vi "UI.vi"() -> ()   [LabVIEW 2017]
panel:
  in  "Run":bool
  in  "Load setting":bool
  in  "stop":bool
  in  "save image":bool
  out "Runtime (ms)":u32
  in  "Save setting":bool
  out "cutting offset":dbl
  out "damaged":dbl
  out "carck":dbl
  out "glitch":dbl
  in  "output folder":path
  out "number":dbl
  in  "input folder":path
  out "display image":T1(plugin-control)
  out "NG code":dbl
  in  "NG_rules":T2
  in  "parameter":T3={"image imshow"=FALSE, "side length (mm)"=0.0, "Main Range (Threshold)"={"Lower value"=73.0, "Upper value"=255.0}, "side velocity threshold"=0.0, "Sub Range (Threshold)"={"Lower value"=73.0, "Upper value"=255.0}, "close kernel size"=0.0, "open kernel size"=0.0, "side angle offest (threshold)"=0.0}
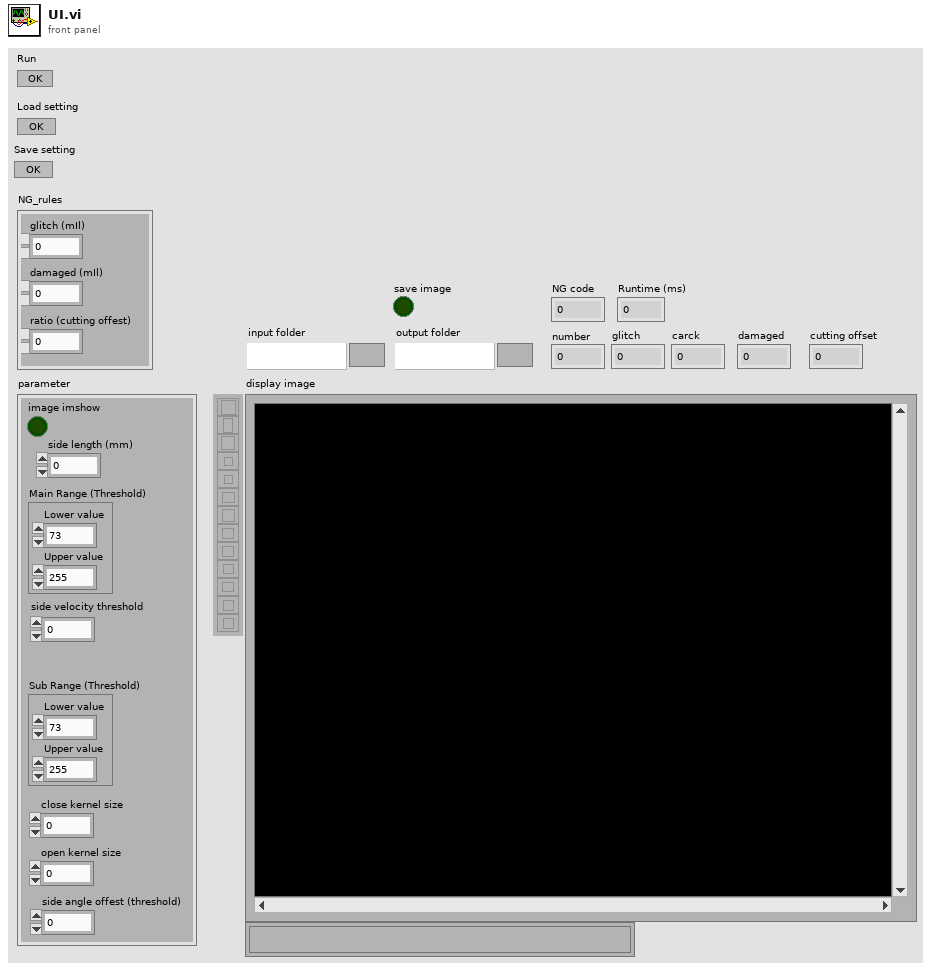
[diagram p1: front panel]
types:
  T1 = typedef "IMAQ Image.ctl" = refnum<image>
  T2 = cluster{"glitch (mIl)":dbl, "damaged (mIl)":dbl, "ratio (cutting offest)":dbl}
  T3 = cluster{"image imshow":bool, "side length (mm)":dbl, "Main Range (Threshold)":cluster{"Lower value":sgl, "Upper value":sgl}, "side velocity threshold":dbl, "Sub Range (Threshold)":cluster{"Lower value":sgl, "Upper value":sgl}, "close kernel size":dbl, "open kernel size":dbl, "side angle offest (threshold)":dbl}
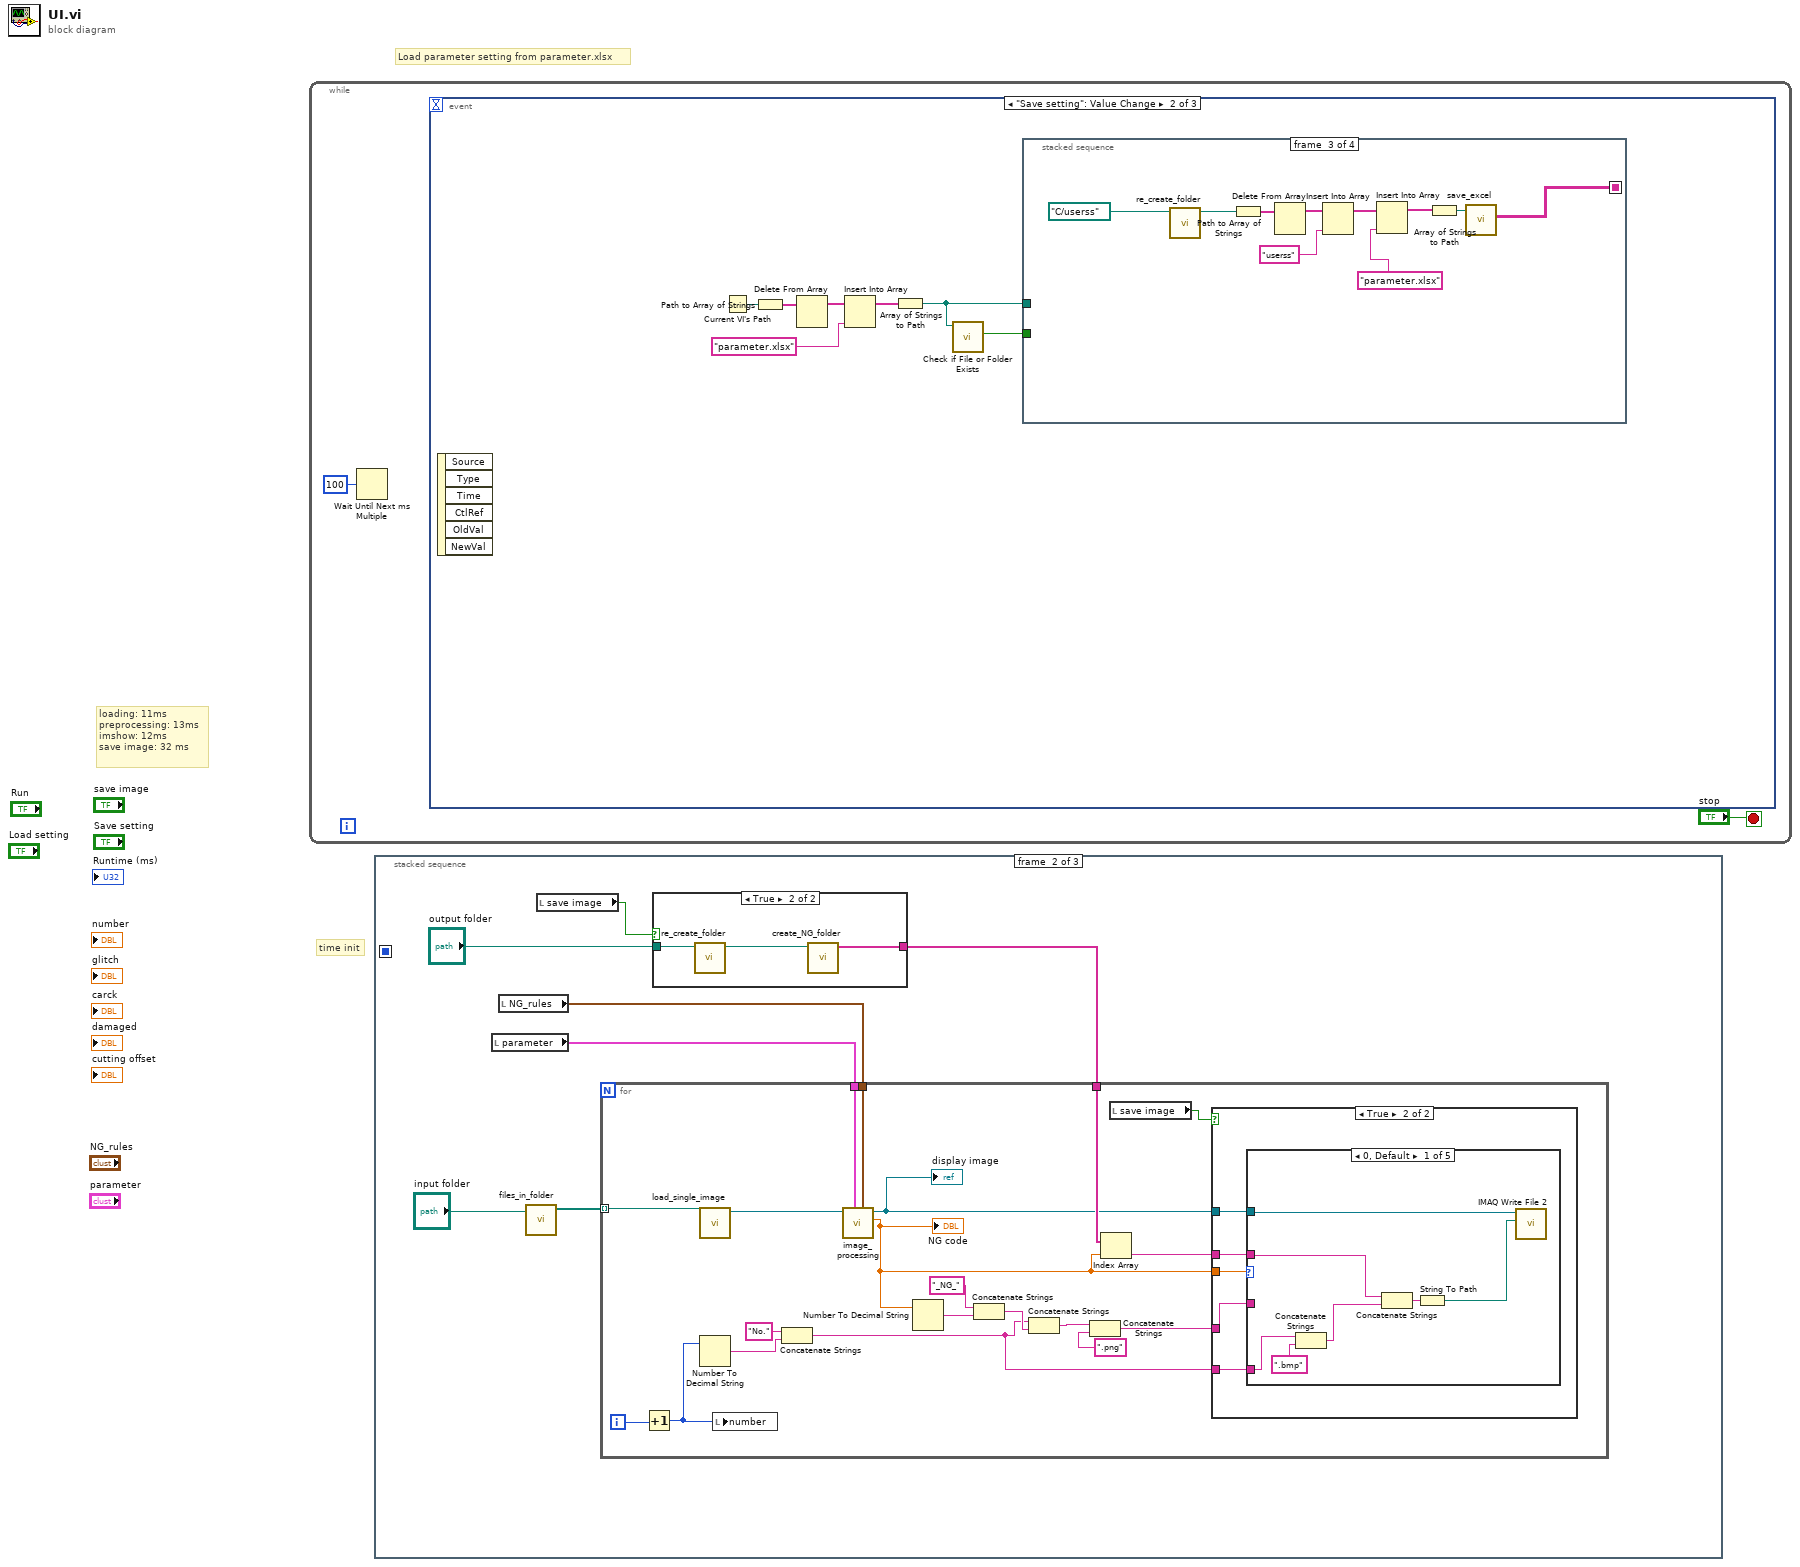
[diagram p0: block diagram]
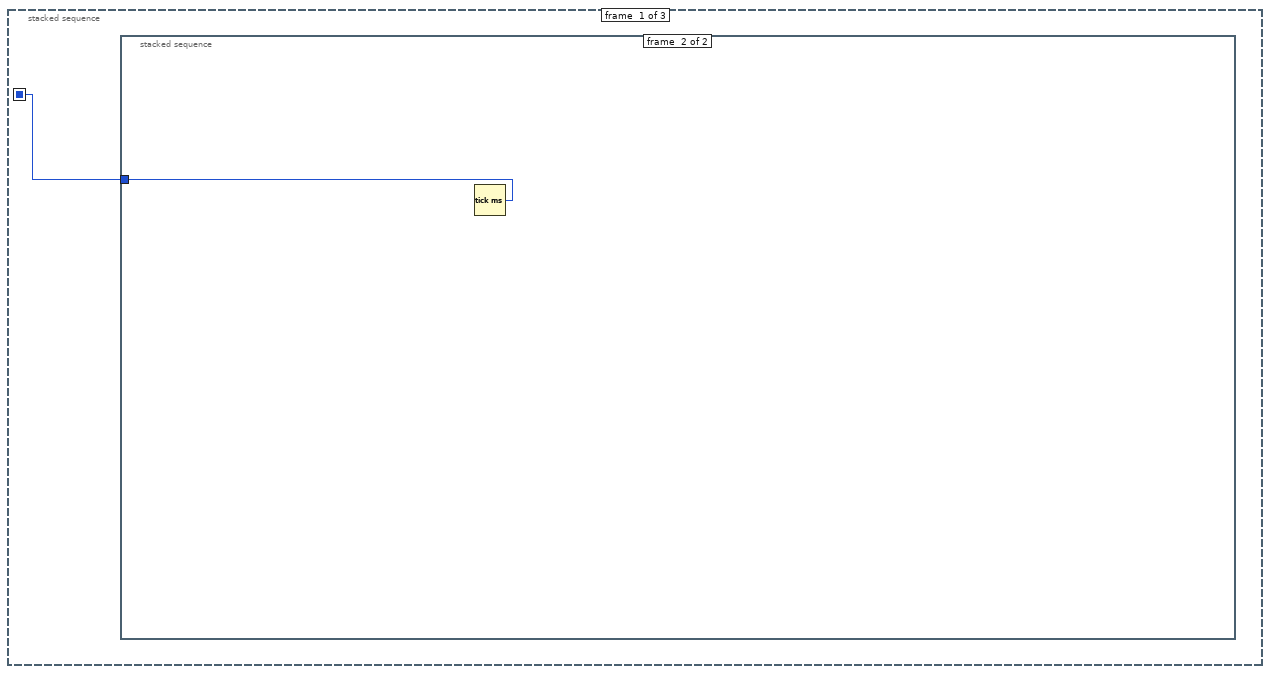
[diagram p2: hidden frame]
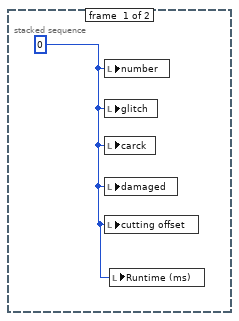
[diagram p3: hidden frame]
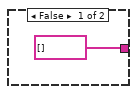
[diagram p4: hidden frame]
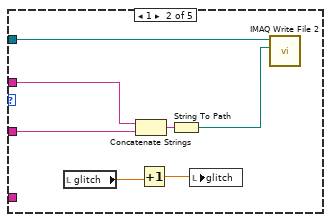
[diagram p6: hidden frame]
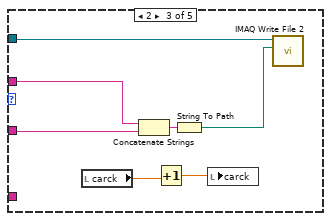
[diagram p7: hidden frame]
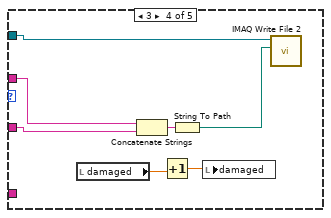
[diagram p8: hidden frame]
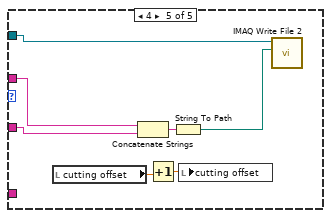
[diagram p9: hidden frame]
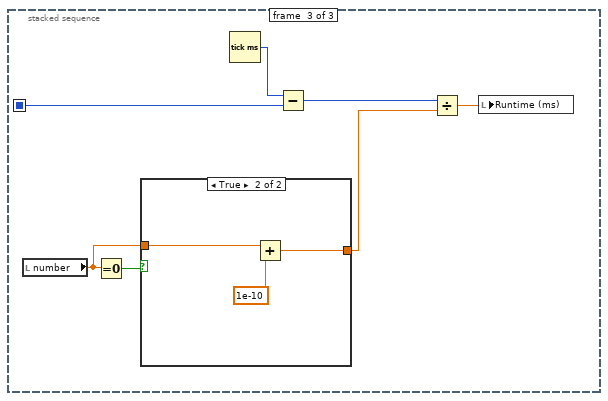
[diagram p10: hidden frame]
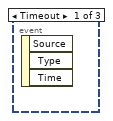
[diagram p12: hidden frame]
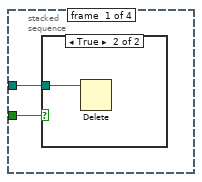
[diagram p13: hidden frame]
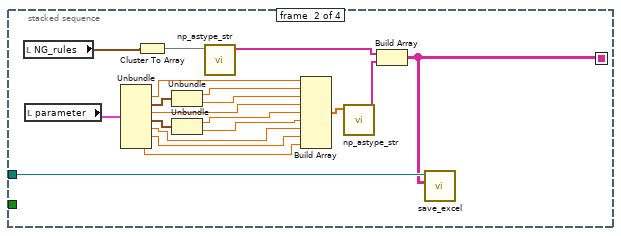
[diagram p15: hidden frame]
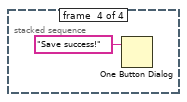
[diagram p16: hidden frame]
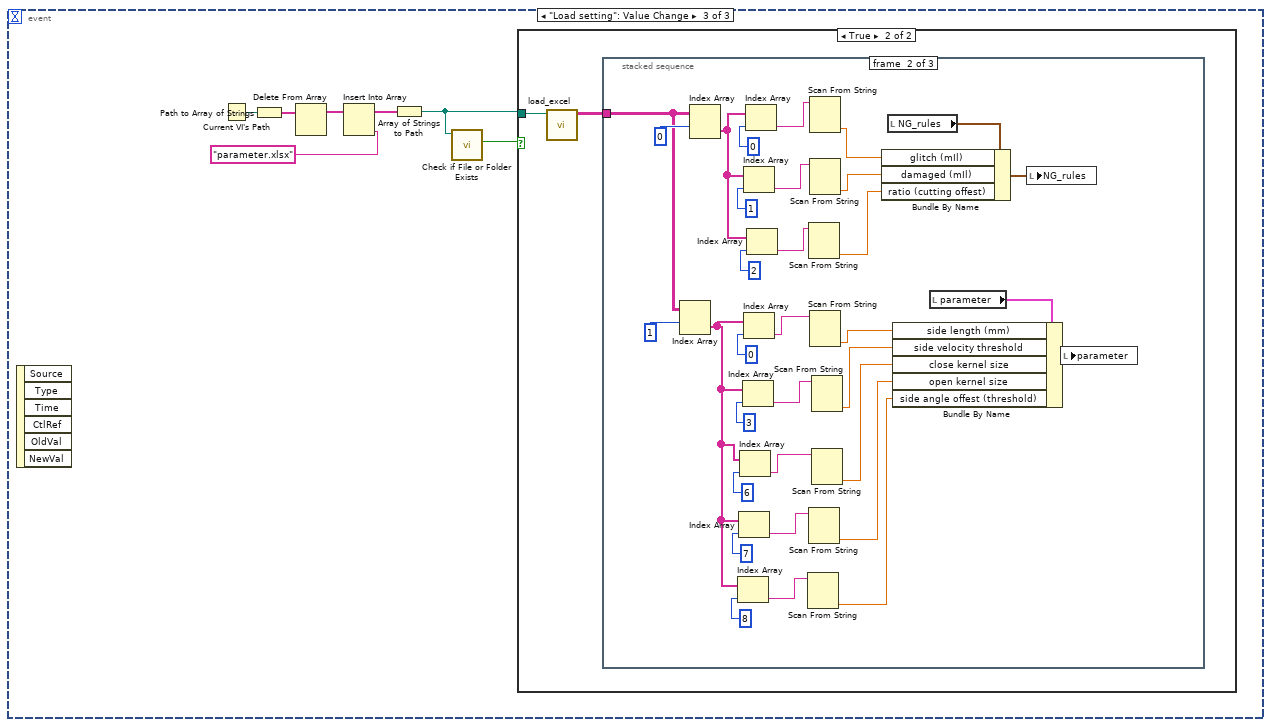
[diagram p17: hidden frame]
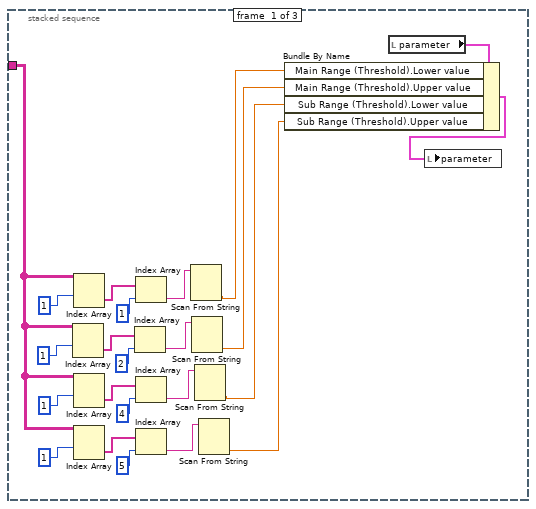
[diagram p19: hidden frame]
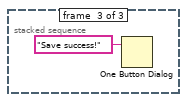
[diagram p20: hidden frame]
diagram:
  # "time init"
  # "loading: 11ms\npreprocessing: 13ms\nimshow: 12ms\nsave image: 32 ms"
  # "Load parameter setting from parameter.xlsx"
  n1 = while {
    stop <- "stop" stop-if-true
    n2 = Wait Until Next ms Multiple(millisecond multiple=u32 100) -> ()  [unwired: 1 out]
    n3 = event shown="[1] \"Save setting\": Value Change" {
      selector: _ -> [_ _ _]
      dyn-events: _ -> [_ _ _]
      timeout: _ -> [_ _ _]
      event Timeout {
        n4 = event-data() -> ()  [unwired: 1 in, 3 out]
      }
      event "Save setting": Value Change {
        n5 = event-data() -> ()  [unwired: 1 in, 6 out]
        n6 = Current VI's Path() -> (path=w7:path)
        n7 = Path to Array of Strings(0:w7) -> (2:w6:string[])  [unwired: 1 out]
        n8 = Delete From Array(array=w6) -> (array with subset deleted=w5:string[])  [unwired: 2 in, 1 out]
        n9 = Insert Into Array(array=w5, new element="parameter.xlsx" ("string")) -> (w4:string[])  [unwired: 1 in]
        n10 = Array of Strings to Path(0:w4) -> (2:w8:path)  [unwired: 1 in]
        n11 = call <vilib>:"Check if File or Folder Exists.vi"("path"=w8) -> ("file or folder exists?"=w9:bool)  [unwired: 8 in, 2 out]
        n12 = stacked-sequence {
          seq-local: [_ w13 _ _] -> [_ _ w41 _]
          tunnel: w8 -> [w11 w18 _ _]
          tunnel: w9 -> [w10 _ _ _]
          frame #0 {
            n13 = case shown="True" w10 {
              tunnel: w11 -> [_ w12]
              frame False {
              }
              frame True {
                n14 = Delete(path (use dialog)=w12) -> ()  [unwired: 4 in, 3 out]
              }
            }
          }
          frame #1 {
            n15 = local read "NG_rules"() -> (w21:T2)
            n16 = local read "parameter"() -> (w31:T3)
            n17 = Unbundle(w31) -> ("side length (mm)"=w28:dbl, "Main Range (Threshold)"=w29:cluster{"Lower value":sgl, "Upper value":sgl}, "side velocity threshold"=w25:dbl, "Sub Range (Threshold)"=w30:cluster{"Lower value":sgl, "Upper value":sgl}, "close kernel size"=w22:dbl, "open kernel size"=w15:dbl, "side angle offest (threshold)"=w14:dbl)  [unwired: 1 out]
            n18 = Cluster To Array(cluster=w21) -> (array=w20:dbl[])
            n19 = Unbundle(w29) -> ("Lower value"=w27:sgl, "Upper value"=w26:sgl)
            n20 = Unbundle(w30) -> ("Lower value"=w24:sgl, "Upper value"=w23:sgl)
            n21 = call "np_astype_str.vi"("NG_rules"=w20) -> ("Array"=w19:string[])  [unwired: 10 in]
            n22 = Build Array(w28, w27, w26, w25, w24, w23, w22, w15, w14) -> (w17:dbl[])
            n23 = call "np_astype_str.vi"("NG_rules"=w17) -> ("Array"=w16:string[])  [unwired: 10 in]
            n24 = Build Array(w19, w16) -> (w13:string[][])
            n25 = call "save_excel.vi"("data in"=w13, "Path"=w18) -> ()  [unwired: 10 in]
          }
          frame #2 {
            n26 = call "re_create_folder.vi"("output folder in"=path "C:/userss") -> ("output folder out"=w36:path)  [unwired: 10 in]
            n27 = Path to Array of Strings(0:w36) -> (2:w39:string[])  [unwired: 1 out]
            n28 = Delete From Array(array=w39) -> (array with subset deleted=w38:string[])  [unwired: 2 in, 1 out]
            n29 = Insert Into Array(array=w38, new element="userss" ("string")) -> (w34:string[])  [unwired: 1 in]
            n30 = Insert Into Array(array=w34, new element="parameter.xlsx" ("string")) -> (w33:string[])  [unwired: 1 in]
            n31 = Array of Strings to Path(0:w33) -> (2:w35:path)  [unwired: 1 in]
            n32 = call "save_excel.vi"("data in"=w41, "Path"=w35) -> ()  [unwired: 10 in]
          }
          frame #3 {
            n33 = One Button Dialog(message="Save success!") -> ()  [unwired: 1 in, 1 out]
          }
        }
      }
      event "Load setting": Value Change {
        n34 = event-data() -> ()  [unwired: 1 in, 6 out]
        n35 = Current VI's Path() -> (path=w46:path)
        n36 = Path to Array of Strings(0:w46) -> (2:w47:string[])  [unwired: 1 out]
        n37 = Delete From Array(array=w47) -> (array with subset deleted=w48:string[])  [unwired: 2 in, 1 out]
        n38 = Insert Into Array(array=w48, new element="parameter.xlsx" ("string")) -> (w49:string[])  [unwired: 1 in]
        n39 = Array of Strings to Path(0:w49) -> (2:w45:path)  [unwired: 1 in]
        n40 = call <vilib>:"Check if File or Folder Exists.vi"("path"=w45) -> ("file or folder exists?"=w44:bool)  [unwired: 8 in, 2 out]
        n41 = case shown="True" w44 {
          tunnel: w45 -> [_ w51]
          frame False {
          }
          frame True {
            n42 = call "load_excel.vi"("Path"=w51) -> ("data"=w50:string[][])  [unwired: 10 in]
            n43 = stacked-sequence {
              tunnel: w50 -> [w60 w99 _]
              frame #0 {
                n44 = Index Array(array=w60, index (row)=1) -> (element=w74:string[])  [unwired: 1 in]
                n45 = Index Array(array=w60, index (row)=1) -> (element=w61:string[])  [unwired: 1 in]
                n46 = Index Array(array=w60, index (row)=1) -> (element=w67:string[])  [unwired: 1 in]
                n47 = Index Array(array=w60, index (row)=1) -> (element=w66:string[])  [unwired: 1 in]
                n48 = Index Array(array=w74, index=2 ("index (row)")) -> (element=w55:string)
                n49 = Index Array(array=w61, index=1 ("index (row)")) -> (element=w54:string)
                n50 = Index Array(array=w67, index=4 ("index (row)")) -> (element=w53:string)
                n51 = Index Array(array=w66, index=5 ("index (row)")) -> (element=w52:string)
                n52 = Scan From String(input string=w54) -> (output 1=w59:dbl)  [unwired: 4 in, 3 out]
                n53 = Scan From String(input string=w55) -> (output 1=w58:dbl)  [unwired: 4 in, 3 out]
                n54 = Scan From String(input string=w53) -> (output 1=w57:dbl)  [unwired: 4 in, 3 out]
                n55 = Scan From String(input string=w52) -> (output 1=w56:dbl)  [unwired: 4 in, 3 out]
                n56 = local read "parameter"() -> (w72:T3)
                n57 = Bundle By Name(cluster=w72, "Main Range (Threshold).Lower value"=w59, "Main Range (Threshold).Upper value"=w58, "Sub Range (Threshold).Lower value"=w57, "Sub Range (Threshold).Upper value"=w56) -> (w71:T3)
                n58 = local write "parameter"(w71) -> ()
              }
              frame #1 {
                n59 = Index Array(array=w99, index (row)=1) -> (element=w75:string[])  [unwired: 1 in]
                n60 = Index Array(array=w99, index (row)=0) -> (element=w101:string[])  [unwired: 1 in]
                n61 = Index Array(array=w75, index=8 ("index (row)")) -> (element=w78:string)
                n62 = Index Array(array=w75, index=7 ("index (row)")) -> (element=w85:string)
                n63 = Index Array(array=w75, index=6 ("index (row)")) -> (element=w86:string)
                n64 = Index Array(array=w75, index=3 ("index (row)")) -> (element=w87:string)
                n65 = Index Array(array=w101, index=1 ("index (row)")) -> (element=w90:string)
                n66 = Index Array(array=w75, index=0 ("index (row)")) -> (element=w88:string)
                n67 = Index Array(array=w101, index=0 ("index (row)")) -> (element=w91:string)
                n68 = Index Array(array=w101, index=2 ("index (row)")) -> (element=w89:string)
                n69 = Scan From String(input string=w78) -> (output 1=w76:dbl)  [unwired: 4 in, 3 out]
                n70 = Scan From String(input string=w89) -> (output 1=w83:dbl)  [unwired: 4 in, 3 out]
                n71 = Scan From String(input string=w85) -> (output 1=w79:dbl)  [unwired: 4 in, 3 out]
                n72 = Scan From String(input string=w91) -> (output 1=w92:dbl)  [unwired: 4 in, 3 out]
                n73 = Scan From String(input string=w90) -> (output 1=w84:dbl)  [unwired: 4 in, 3 out]
                n74 = Scan From String(input string=w88) -> (output 1=w82:dbl)  [unwired: 4 in, 3 out]
                n75 = Scan From String(input string=w87) -> (output 1=w81:dbl)  [unwired: 4 in, 3 out]
                n76 = Scan From String(input string=w86) -> (output 1=w80:dbl)  [unwired: 4 in, 3 out]
                n77 = local read "NG_rules"() -> (w102:T2)
                n78 = Bundle By Name(cluster=w102, "glitch (mIl)"=w92, "damaged (mIl)"=w84, "ratio (cutting offest)"=w83) -> (w105:T2)
                n79 = local read "parameter"() -> (w93:T3)
                n80 = Bundle By Name(cluster=w93, "side length (mm)"=w82, "side velocity threshold"=w81, "close kernel size"=w80, "open kernel size"=w79, "side angle offest (threshold)"=w76) -> (w97:T3)
                n81 = local write "NG_rules"(w105) -> ()
                n82 = local write "parameter"(w97) -> ()
              }
              frame #2 {
                n83 = One Button Dialog(message="Save success!") -> ()  [unwired: 1 in, 1 out]
              }
            }
          }
        }
      }
    }
  }
  n84 = stacked-sequence {
    seq-local: [w109 _ _] -> [_ _ w188]
    frame #0 {
      n85 = stacked-sequence {
        tunnel: [_ w111] -> w109
        frame #0 {
          w110 = 0
          n86 = local write "number"(w110) -> ()
          n87 = local write "glitch"(w110) -> ()
          n88 = local write "carck"(w110) -> ()
          n89 = local write "damaged"(w110) -> ()
          n90 = local write "cutting offset"(w110) -> ()
          n91 = local write "Runtime (ms)"(w110) -> ()
        }
        frame #1 {
          n92 = Tick Count (ms)() -> (millisecond timer value=w111:u32)
        }
      }
    }
    frame #1 {
      n93 = local read "parameter"() -> (w114:T3)
      n94 = local read "NG_rules"() -> (w113:T2)
      n95 = call "files_in_folder.vi"("folder path"="input folder") -> ("Array"=w116:path[])  [unwired: 10 in]
      n96 = local read "save image"() -> (w112:bool)
      n97 = case shown="True" w112 {
        tunnel: "output folder" -> [_ w122]
        tunnel: [string[] [] ("NG folder array") w120] -> w115
        frame False {
        }
        frame True {
          n98 = call "re_create_folder.vi"("output folder in"=w122) -> ("output folder out"=w121:path)  [unwired: 10 in]
          n99 = call "create_NG_folder.vi"("output folder in"=w121) -> ("NG folder array"=w120:string[])  [unwired: 10 in]
        }
      }
      n100 = for {
        tunnel: w113 -> [w142]
        tunnel: w114 -> [w123]
        tunnel: w116 -> [w140] mode=indexing
        tunnel: w115 -> [w129]
        i -> [w137]
        n101 = Increment(x=w137) -> (x+1=w130:i32)
        n102 = call "load_single_image.vi"("Path"=w140) -> ("Refnum out"=w141:T1)  [unwired: 10 in]
        n103 = Number To Decimal String(number=w130) -> (decimal integer string=w133:string)  [unwired: 1 in]
        n104 = local write "number"(w130) -> ()
        n105 = Concatenate Strings("No." ("string"), w133) -> (w126:string)
        n106 = call "image_processing.vi"("NG_rules"=w142, "parameter"=w123, "image"=w141) -> ("NG code"=w128:dbl, "display image"=w124:T1)  [unwired: 6 in, 1 out]
        "NG code" <- w128
        "display image" <- w124
        n107 = Number To Decimal String(number=w128) -> (decimal integer string=w136:string)  [unwired: 1 in]
        n108 = Concatenate Strings("_NG_" ("string"), w136) -> (w131:string)
        n109 = Concatenate Strings(w126, w131) -> (w132:string)
        n110 = Concatenate Strings(w132, ".png" ("string")) -> (w138:string)
        n111 = Index Array(array=w129, index=w128) -> (element=w127:string)
        n112 = local read "save image"() -> (w125:bool)
        n113 = case shown="True" w125 {
          tunnel: w124 -> [_ w147]
          tunnel: w138 -> [_ w146]
          tunnel: w128 -> [_ w143]
          tunnel: w127 -> [_ w145]
          tunnel: w126 -> [_ w144]
          frame False {
          }
          frame True {
            n114 = case shown="0, Default" w143 {
              tunnel: w147 -> [w152 w161 w165 w173 w180]
              tunnel: w146 -> [_ w158 w166 w172 w179]
              tunnel: w145 -> [w151 w155 w162 w169 w176]
              tunnel: w144 -> [w150 _ _ _ _]
              frame 0, Default {
                n115 = Concatenate Strings(w150, ".bmp" ("string")) -> (w148:string)
                n116 = Concatenate Strings(w151, w148) -> (w153:string)
                n117 = String To Path(string=w153) -> (path=w154:path)
                n118 = call-poly "IMAQ Write File 2"("File Path"=w154, "Image"=w152) -> ()  [unwired: 8 in, 2 out]
              }
              frame 1 {
                n119 = local read "glitch"() -> (w157:dbl)
                n120 = Concatenate Strings(w155, w158) -> (w159:string)
                n121 = Increment(x=w157) -> (x+1=w156:dbl)
                n122 = String To Path(string=w159) -> (path=w160:path)
                n123 = local write "glitch"(w156) -> ()
                n124 = call-poly "IMAQ Write File 2"("File Path"=w160, "Image"=w161) -> ()  [unwired: 8 in, 2 out]
              }
              frame 2 {
                n125 = local read "carck"() -> (w164:dbl)
                n126 = Concatenate Strings(w162, w166) -> (w167:string)
                n127 = Increment(x=w164) -> (x+1=w163:dbl)
                n128 = String To Path(string=w167) -> (path=w168:path)
                n129 = local write "carck"(w163) -> ()
                n130 = call-poly "IMAQ Write File 2"("File Path"=w168, "Image"=w165) -> ()  [unwired: 8 in, 2 out]
              }
              frame 3 {
                n131 = local read "damaged"() -> (w171:dbl)
                n132 = Concatenate Strings(w169, w172) -> (w174:string)
                n133 = Increment(x=w171) -> (x+1=w170:dbl)
                n134 = String To Path(string=w174) -> (path=w175:path)
                n135 = local write "damaged"(w170) -> ()
                n136 = call-poly "IMAQ Write File 2"("File Path"=w175, "Image"=w173) -> ()  [unwired: 8 in, 2 out]
              }
              frame 4 {
                n137 = local read "cutting offset"() -> (w178:dbl)
                n138 = Concatenate Strings(w176, w179) -> (w181:string)
                n139 = Increment(x=w178) -> (x+1=w177:dbl)
                n140 = String To Path(string=w181) -> (path=w182:path)
                n141 = local write "cutting offset"(w177) -> ()
                n142 = call-poly "IMAQ Write File 2"("File Path"=w182, "Image"=w180) -> ()  [unwired: 8 in, 2 out]
              }
            }
          }
        }
      }
    }
    frame #2 {
      n143 = local read "number"() -> (w184:dbl)
      n144 = Equal To 0?(x=w184) -> (x = 0?=w186:bool)
      n145 = case shown="True" w186 {
        tunnel: [w190 w192] -> w185
        tunnel: w184 -> [w190 w191]
        frame False {
        }
        frame True {
          n146 = Add(x=w191, y=1e-10) -> (x+y=w192:dbl)
        }
      }
      n147 = Tick Count (ms)() -> (millisecond timer value=w189:u32)
      n148 = Subtract(x=w189, y=w188) -> (x-y=w187:u32)
      n149 = Divide(x=w187, y=w185) -> (x/y=w183:dbl)
      n150 = local write "Runtime (ms)"(w183) -> ()
    }
  }
